vi "VrmVISACheckResponse.vi"(8 "error in (no error)":errorcluster, 10 "Response":string) -> (0 "error out":errorcluster, 2 "Response out":string)   [LabVIEW 2021]
uses:
  <vilib>/regexp/Match Regular Expression.xnode
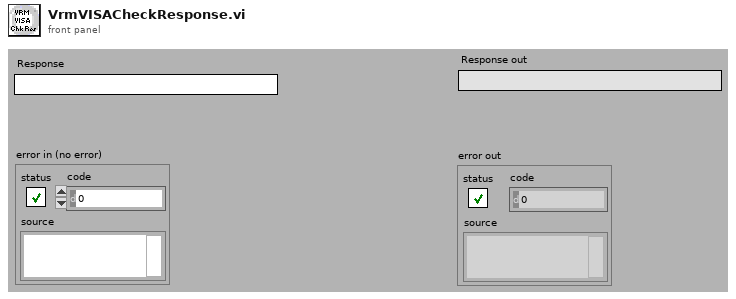
[diagram p1: front panel]
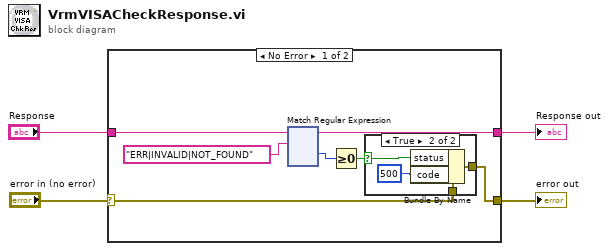
[diagram p0: block diagram]
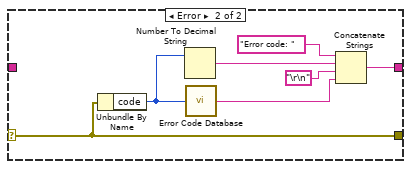
[diagram p3: hidden frame]
diagram:
  n1 = case shown="No Error" "error in (no error)" {
    selector: "error in (no error)" -> [w8 w139]
    tunnel: "Response" -> [w6 _]
    tunnel: [w9 w139] -> w2
    tunnel: [w6 w134] -> w1
    frame No Error {
      n2 = xnode "Match Regular Expression"("input string"=w6, "regular expression"="ERR|INVALID|NOT_FOUND") -> ("offset past match"=w7:i32)  [unwired: 4 in, 4 out]
      n3 = Greater Or Equal To 0?(x=w7) -> (x >= 0?=w5:bool)
      n4 = case shown="True" w5 {
        selector: w5 -> [_ w13]
        tunnel: [w11 w15] -> w9
        tunnel: w8 -> [w11 w14]
        frame False {
        }
        frame True {
          n5 = Bundle By Name(cluster=w14, "status"=w13, "code"=500) -> (w15:errorcluster)
        }
      }
    }
    frame Error {
      n6 = Unbundle By Name(w139) -> ("code"=w138:i32)
      n7 = Number To Decimal String(number=w138) -> (decimal integer string=w137:string)  [unwired: 1 in]
      n8 = call <vilib>:"Error Code Database.vi"("Error Code"=w138) -> ("Error Text"=w135:string)
      n9 = Concatenate Strings("Error code: " ("string"), w137, "\r\n", w135) -> (w134:string)
    }
  }
  "Response out" <- w1
  "error out" <- w2
